vi "HSVtoRGB.vi"(9 "Value":dbl, 10 "Saturation":dbl=1.0, 11 "Hue [0,1)":dbl) -> (1 "Blue":u8, 2 "Green":u8, 3 "Red":u8)   [LabVIEW 2016]
doc: "Convert HSV to RGB Values. H is expressed as a value from 0-1, rather than 0-360. \n\n0= < H < 1"
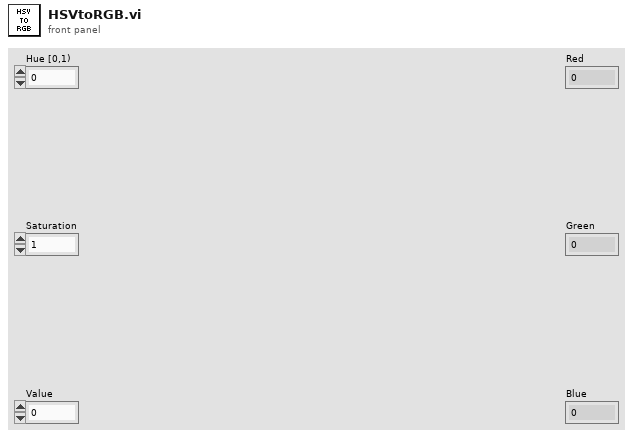
[diagram p1: front panel]
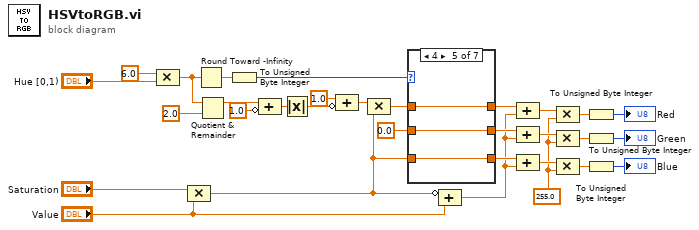
[diagram p0: block diagram]
diagram:
  w3 = 255.0 ("y")
  n1 = Compound Arithmetic op=MULTIPLY(6.0 ("y"), "Hue [0,1)") -> (w4:dbl)
  n2 = Compound Arithmetic op=MULTIPLY("Saturation", "Value") -> (w1:dbl)
  n3 = Round Toward -Infinity(1:w4) -> (0:w27:dbl)
  n4 = Quotient & Remainder(x=w4, y=2.0) -> (x-y*floor(x/y)=w12:dbl)  [unwired: 1 out]
  n5 = To Unsigned Byte Integer(number=w27) -> (unsigned 8bit integer=w14:u8)
  n6 = Compound Arithmetic op=ADD(w12, invert 1.0 ("y")) -> (w10:dbl)
  n7 = Absolute Value(x=w10) -> (abs(x)=w9:dbl)
  n8 = Compound Arithmetic op=ADD(1.0 ("x"), invert w9) -> (w7:dbl)
  n9 = Compound Arithmetic op=MULTIPLY(w7, w1) -> (w26:dbl)
  n10 = case shown="4" w14 {
    tunnel: w1 -> [w34 w36 w39 w43 w44 w49 _]
    tunnel: w26 -> [w33 w37 w38 w42 w46 w47 _]
    tunnel: 0.0 -> [w32 w35 w40 w41 w45 w48 w50]
    tunnel: [w34 w37 w40 w41 w46 w49 w50] -> w22
    tunnel: [w33 w36 w39 w42 w45 w48 w50] -> w23
    tunnel: [w32 w35 w38 w43 w44 w47 w50] -> w24
    frame 0 {
    }
    frame 1 {
    }
    frame 2 {
    }
    frame 3 {
    }
    frame 4 {
    }
    frame 5 {
    }
    frame Default {
    }
  }
  n11 = Compound Arithmetic op=ADD(invert w1, "Value") -> (w21:dbl)
  n12 = Compound Arithmetic op=ADD(w22, w21) -> (w15:dbl)
  n13 = Compound Arithmetic op=ADD(w23, w21) -> (w16:dbl)
  n14 = Compound Arithmetic op=ADD(w24, w21) -> (w17:dbl)
  n15 = Compound Arithmetic op=MULTIPLY(w15, w3) -> (w20:dbl)
  n16 = Compound Arithmetic op=MULTIPLY(w16, w3) -> (w19:dbl)
  n17 = Compound Arithmetic op=MULTIPLY(w17, w3) -> (w18:dbl)
  n18 = To Unsigned Byte Integer(number=w20) -> (unsigned 8bit integer=→"Red":u8)
  n19 = To Unsigned Byte Integer(number=w19) -> (unsigned 8bit integer=→"Green":u8)
  n20 = To Unsigned Byte Integer(number=w18) -> (unsigned 8bit integer=→"Blue":u8)
